vi "Calc SIM Inputs.vi"(7 "time (s)":dbl, 9 "SIM INI":T1, 10 "uIC":dbl[](array[numeric]), 11 "SIM Init":T2) -> (3 "SIM Inputs":T4)   [LabVIEW 2015]
uses:
  typedefs/sim inputs.ctl
  typedefs/init data.ctl
  typedefs/SIM type.ctl
  SIM INI.ctl
  <vilib>/Utility/inputDevices.llb/joystickAcquire.vi
  <vilib>/express/express arith-compare/Formula/XNode/ExpressFormulaBlockNode.xnode
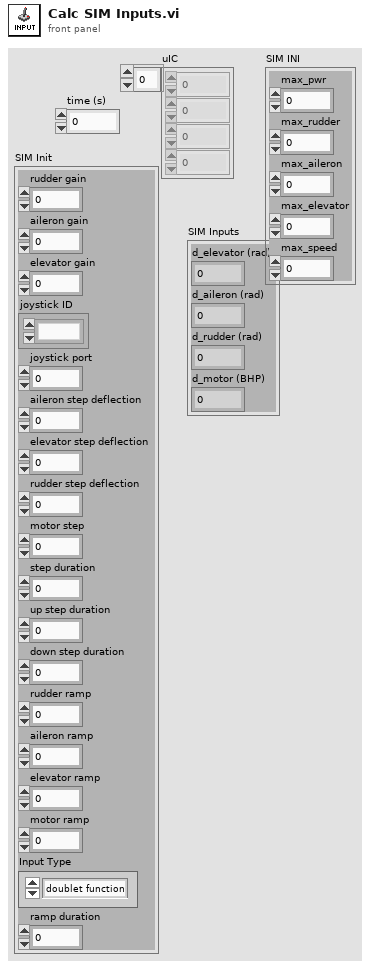
[diagram p1: front panel]
types:
  T1 = typedef "SIM INI.ctl" = cluster{"max_pwr":dbl, "max_rudder":dbl, "max_aileron":dbl, "max_elevator":dbl, "max_speed":dbl}
  T2 = typedef "init data.ctl" = cluster{"rudder gain":dbl, "aileron gain":dbl, "elevator gain":dbl, "joystick ID":refnum<k1>, "joystick port":i32, "aileron step deflection":dbl, "elevator step deflection":dbl, "rudder step deflection":dbl, "motor step":dbl, "step duration":dbl, "up step duration":dbl, "down step duration":dbl, "rudder ramp":dbl, "aileron ramp":dbl, "elevator ramp":dbl, "motor ramp":dbl, "Input Type":T3, "ramp duration":dbl}
  T3 = typedef "SIM type.ctl" = enum16{"doublet function", "ramp function", "step function", "joystick (select port)", "joystick (autodetect)"}
  T4 = typedef "sim inputs.ctl" = cluster{"d_elevator (rad)":dbl, "d_aileron (rad)":dbl, "d_rudder (rad)":dbl, "d_motor (BHP)":dbl}
  T5 = cluster{"X axis":i32, "Y axis":i32, "Z axis":i32, "X axis rotation":i32, "Y axis rotation":i32, "Z axis rotation":i32, "U axis":i32, "V axis":i32}
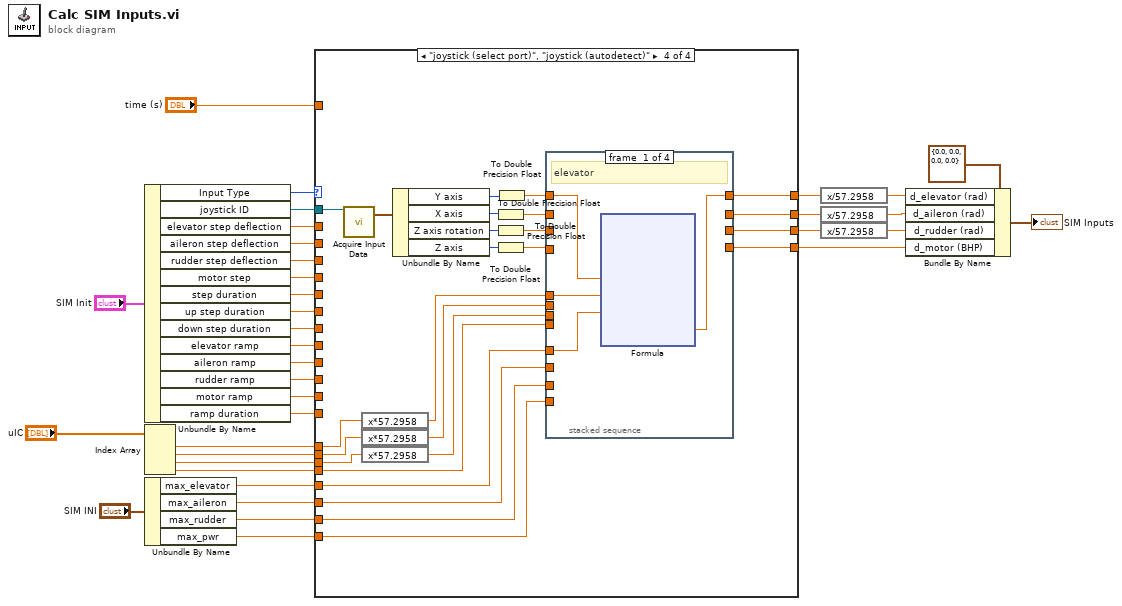
[diagram p0: block diagram]
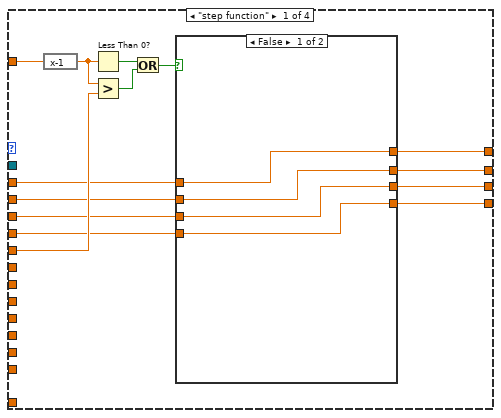
[diagram p2: hidden frame]
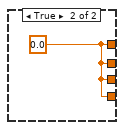
[diagram p3: hidden frame]
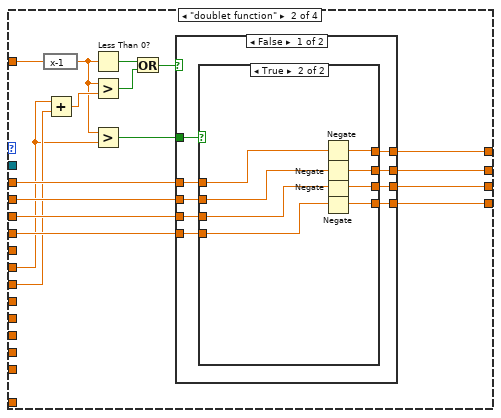
[diagram p4: hidden frame]
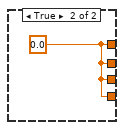
[diagram p6: hidden frame]
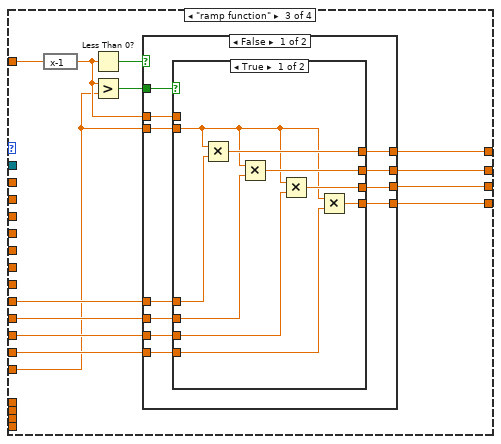
[diagram p7: hidden frame]
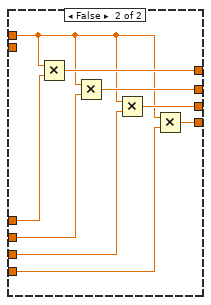
[diagram p8: hidden frame]
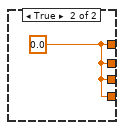
[diagram p9: hidden frame]
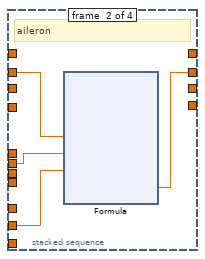
[diagram p10: hidden frame]
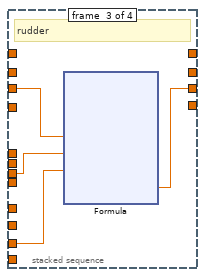
[diagram p11: hidden frame]
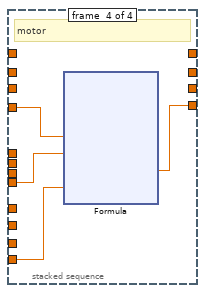
[diagram p12: hidden frame]
diagram:
  n1 = Unbundle By Name("SIM Init") -> ("Input Type"=w34:T3, "joystick ID"=w33:refnum<k1>, "elevator step deflection"=w28:dbl, "aileron step deflection"=w27:dbl, "rudder step deflection"=w26:dbl, "motor step"=w25:dbl, "step duration"=w24:dbl, "up step duration"=w23:dbl, "down step duration"=w22:dbl, "elevator ramp"=w21:dbl, "aileron ramp"=w20:dbl, "rudder ramp"=w19:dbl, "motor ramp"=w18:dbl, "ramp duration"=w17:dbl)
  n2 = Index Array(array="uIC") -> (element #1=w10:dbl, element #2=w9:dbl, element #3=w8:dbl, element #4=w7:dbl)  [unwired: 4 in]
  n3 = Unbundle By Name("SIM INI") -> ("max_elevator"=w15:dbl, "max_aileron"=w14:dbl, "max_rudder"=w13:dbl, "max_pwr"=w12:dbl)
  n4 = case shown="\"joystick (select port)\", \"joystick (autodetect)\"" w34 {
    tunnel: w33 -> [_ _ _ w156]
    tunnel: [w36 w60 w103 w144] -> w31
    tunnel: [w37 w61 w104 w145] -> w4
    tunnel: [w38 w62 w105 w146] -> w5
    tunnel: [w39 w63 w106 w147] -> w6
    tunnel: "time (s)" -> [w49 w71 w97 _]
    tunnel: w28 -> [w43 w67 _ _]
    tunnel: w27 -> [w42 w66 _ _]
    tunnel: w26 -> [w41 w65 _ _]
    tunnel: w25 -> [w40 w64 _ _]
    tunnel: w24 -> [w46 _ _ _]
    tunnel: w23 -> [_ w56 _ _]
    tunnel: w22 -> [_ w59 _ _]
    tunnel: w21 -> [_ _ w98 _]
    tunnel: w20 -> [_ _ w99 _]
    tunnel: w19 -> [_ _ w100 _]
    tunnel: w18 -> [_ _ w101 _]
    tunnel: w17 -> [_ _ w94 _]
    tunnel: w15 -> [_ _ _ w151]
    tunnel: w14 -> [_ _ _ w150]
    tunnel: w13 -> [_ _ _ w149]
    tunnel: w12 -> [_ _ _ w148]
    tunnel: w10 -> [_ _ _ w143]
    tunnel: w9 -> [_ _ _ w141]
    tunnel: w8 -> [_ _ _ w142]
    tunnel: w7 -> [_ _ _ w137]
    frame "step function" {
      n5 = expression code="x-1"(w49) -> (w47:dbl)
      n6 = Less Than 0?(x=w47) -> (x < 0?=w48:bool)
      n7 = Greater?(x=w47, y=w46) -> (0:w45:bool)
      n8 = Or(x=w48, y=w45) -> (x .or. y?=w44:bool)
      n9 = case shown="False" w44 {
        tunnel: w43 -> [w53 _]
        tunnel: w42 -> [w52 _]
        tunnel: w41 -> [w51 _]
        tunnel: w40 -> [w50 _]
        tunnel: [w53 w54] -> w39
        tunnel: [w52 w54] -> w38
        tunnel: [w51 w54] -> w37
        tunnel: [w50 w54] -> w36
        frame False {
        }
        frame True {
          w54 = 0.0 ("aileron step deflection")
        }
      }
    }
    frame "doublet function" {
      n10 = expression code="x-1"(w71) -> (w57:dbl)
      n11 = Add(x=w56, y=w59) -> (x+y=w58:dbl)
      n12 = Less Than 0?(x=w57) -> (x < 0?=w70:bool)
      n13 = Greater?(x=w57, y=w58) -> (0:w69:bool)
      n14 = Greater?(x=w57, y=w56) -> (0:w55:bool)
      n15 = Or(x=w70, y=w69) -> (x .or. y?=w68:bool)
      n16 = case shown="False" w68 {
        tunnel: w67 -> [w78 _]
        tunnel: w66 -> [w76 _]
        tunnel: w65 -> [w74 _]
        tunnel: w64 -> [w72 _]
        tunnel: [w79 w93] -> w63
        tunnel: [w77 w93] -> w62
        tunnel: [w75 w93] -> w61
        tunnel: [w73 w93] -> w60
        tunnel: w55 -> [w80 _]
        frame False {
          n17 = case shown="True" w80 {
            tunnel: [w84 w92] -> w79
            tunnel: w78 -> [w84 w85]
            tunnel: [w83 w91] -> w77
            tunnel: w76 -> [w83 w86]
            tunnel: [w82 w90] -> w75
            tunnel: w74 -> [w82 w87]
            tunnel: [w81 w89] -> w73
            tunnel: w72 -> [w81 w88]
            frame False {
            }
            frame True {
              n18 = Negate(x=w85) -> (-x=w92:dbl)
              n19 = Negate(x=w86) -> (-x=w91:dbl)
              n20 = Negate(x=w87) -> (-x=w90:dbl)
              n21 = Negate(x=w88) -> (-x=w89:dbl)
            }
          }
        }
        frame True {
          w93 = 0.0 ("aileron step deflection")
        }
      }
    }
    frame "ramp function" {
      n22 = expression code="x-1"(w97) -> (w96:dbl)
      n23 = Less Than 0?(x=w96) -> (x < 0?=w102:bool)
      n24 = Greater?(x=w96, y=w94) -> (0:w95:bool)
      n25 = case shown="False" w102 {
        tunnel: [w117 w136] -> w106
        tunnel: [w116 w136] -> w105
        tunnel: [w115 w136] -> w104
        tunnel: [w114 w136] -> w103
        tunnel: w101 -> [w109 _]
        tunnel: w100 -> [w110 _]
        tunnel: w99 -> [w111 _]
        tunnel: w98 -> [w112 _]
        tunnel: w96 -> [w113 _]
        tunnel: w95 -> [w108 _]
        tunnel: w94 -> [w107 _]
        frame False {
          n26 = case shown="True" w108 {
            tunnel: [w126 w135] -> w117
            tunnel: [w125 w134] -> w116
            tunnel: [w124 w133] -> w115
            tunnel: [w123 w132] -> w114
            tunnel: w113 -> [_ w131]
            tunnel: w112 -> [w122 w130]
            tunnel: w111 -> [w121 w129]
            tunnel: w110 -> [w120 w128]
            tunnel: w109 -> [w119 w127]
            tunnel: w107 -> [w118 _]
            frame True {
              n27 = Multiply(x=w118, y=w122) -> (x*y=w126:dbl)
              n28 = Multiply(x=w118, y=w121) -> (x*y=w125:dbl)
              n29 = Multiply(x=w118, y=w120) -> (x*y=w124:dbl)
              n30 = Multiply(x=w118, y=w119) -> (x*y=w123:dbl)
            }
            frame False {
              n31 = Multiply(x=w131, y=w130) -> (x*y=w135:dbl)
              n32 = Multiply(x=w131, y=w129) -> (x*y=w134:dbl)
              n33 = Multiply(x=w131, y=w128) -> (x*y=w133:dbl)
              n34 = Multiply(x=w131, y=w127) -> (x*y=w132:dbl)
            }
          }
        }
        frame True {
          w136 = 0.0 ("aileron step deflection")
        }
      }
    }
    frame "joystick (select port)", "joystick (autodetect)" {
      n35 = call-poly <vilib>:"Acquire Input Data.vi"("device ID"=w156) -> ("axis info"=w158:T5)  [unwired: 14 in, 4 out]
      n36 = expression code="x*57.2958"(w143) -> (w140:dbl)
      n37 = expression code="x*57.2958"(w141) -> (w139:dbl)
      n38 = expression code="x*57.2958"(w142) -> (w138:dbl)
      n39 = Unbundle By Name(w158) -> ("Y axis"=w157:i32, "X axis"=w159:i32, "Z axis rotation"=w160:i32, "Z axis"=w161:i32)
      n40 = To Double Precision Float(number=w159) -> (double precision float=w154:dbl)
      n41 = To Double Precision Float(number=w160) -> (double precision float=w153:dbl)
      n42 = To Double Precision Float(number=w161) -> (double precision float=w152:dbl)
      n43 = To Double Precision Float(number=w157) -> (double precision float=w155:dbl)
      n44 = stacked-sequence {
        tunnel: w155 -> [w165 _ _ _]
        tunnel: w154 -> [_ w181 _ _]
        tunnel: w153 -> [_ _ w197 _]
        tunnel: w152 -> [_ _ _ w213]
        tunnel: w151 -> [w164 _ _ _]
        tunnel: w150 -> [_ w180 _ _]
        tunnel: w149 -> [_ _ w196 _]
        tunnel: w148 -> [_ _ _ w212]
        tunnel: [w163 _ _ _] -> w147
        tunnel: [_ w179 _ _] -> w146
        tunnel: [_ _ w195 _] -> w145
        tunnel: [_ _ _ w211] -> w144
        tunnel: w140 -> [w162 _ _ _]
        tunnel: w139 -> [_ w178 _ _]
        tunnel: w138 -> [_ _ w194 _]
        tunnel: w137 -> [_ _ _ w210]
        frame #0 {
          # "elevator"
          n45 = xnode "Formula"("input"=w165, "Trim"=w162, "Max"=w164) -> ("Result"=w163:dbl)  [unwired: 1 in, 1 out]
        }
        frame #1 {
          # "aileron"
          n46 = xnode "Formula"("input"=w181, "Trim"=w178, "Max"=w180) -> ("Result"=w179:dbl)  [unwired: 1 in, 1 out]
        }
        frame #2 {
          # "rudder"
          n47 = xnode "Formula"("input"=w197, "Trim"=w194, "Max"=w196) -> ("Result"=w195:dbl)  [unwired: 1 in, 1 out]
        }
        frame #3 {
          # "motor"
          n48 = xnode "Formula"("input"=w213, "Trim"=w210, "Max"=w212) -> ("Result"=w211:dbl)  [unwired: 1 in, 1 out]
        }
      }
    }
  }
  n49 = expression code="x/57.2958"(w6) -> (w3:dbl)
  n50 = expression code="x/57.2958"(w5) -> (w2:dbl)
  n51 = expression code="x/57.2958"(w4) -> (w1:dbl)
  n52 = Bundle By Name(cluster=T4 {"d_elevator (rad)"=0.0, "d_aileron (rad)"=0.0, "d_rudder (rad)"=0.0, "d_motor (BHP)"=0.0} ("SIM Inputs"), "d_elevator (rad)"=w3, "d_aileron (rad)"=w2, "d_rudder (rad)"=w1, "d_motor (BHP)"=w31) -> (→"SIM Inputs":T4)
